vi "FL_Reshape_data_for_memory_storage.vi"(11 "DEC SGL input":sgl[][](array[numeric])) -> (3 "DEC SGL Output":sgl[](array[numeric]))   [LabVIEW 2016]
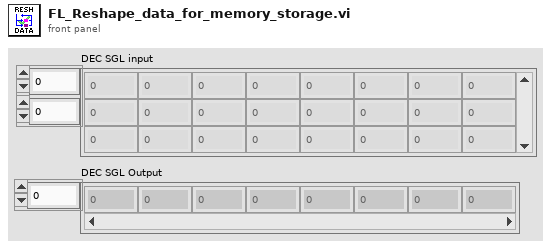
[diagram p1: front panel]
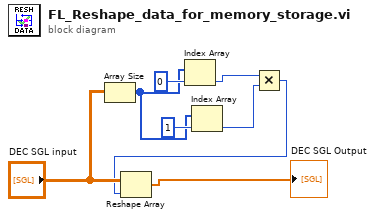
[diagram p0: block diagram]
diagram:
  n1 = Array Size(array="DEC SGL input") -> (size(s)=w4:i32[])
  n2 = Index Array(array=w4, index=0) -> (element=w3:i32)
  n3 = Index Array(array=w4, index=1) -> (element=w2:i32)
  n4 = Multiply(x=w3, y=w2) -> (x*y=w1:i32)
  n5 = Reshape Array("DEC SGL input", w1) -> (→"DEC SGL Output":sgl[])
